vi "Test Attach Debugger.vi"   [LabVIEW 2020, in "Test Process.lvclass"]
uses:
  Test Process.lvclass
  C:/Program Files (x86)/National Instruments/LabVIEW 2020/vi.lib/Astemes/Triarc Framework/Process/Process.lvclass
  <vilib>/Astemes/Triarc Framework/Process/Process.lvclass/Process.ctl
  <vilib>/Astemes/Triarc Framework/Process/Private/SubVIs/Wait for finish.vi
  <vilib>/Astemes/Triarc Framework/Process/Protected/Messaging/Enqueue Message.vi
  <vilib>/Astemes/Triarc Framework/Process/Private/SubVIs/Set Lifecycle State.vi
  <vilib>/Astemes/Triarc Framework/Process/Public/Lifecycle/Get Lifecycle State.vi
  <vilib>/Astemes/Triarc Framework/Process/Private/SubVIs/Handle Debug Data.vi
  <vilib>/Utility/error.llb/Clear Errors.vi
  <vilib>/Astemes/Triarc Framework/Logging/Log Debug.vi
  <vilib>/AdvancedString/1D String Array to Delimited String.vi
  <vilib>/Utility/High Resolution Relative Seconds.vi
  <vilib>/Utility/error.llb/Error Cluster From Error Code.vi
  <vilib>/Astemes/Triarc Framework/Process/Public/Read Name.vi
  <vilib>/Astemes/Triarc Framework/Process/Process.lvclass
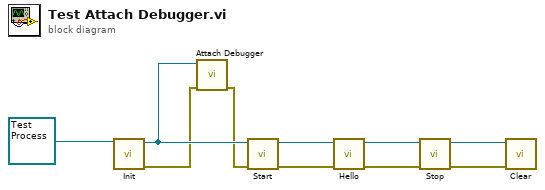
[diagram p0: block diagram]
diagram:
  n1 = call-dynamic "Init.vi"("Process In"=refnum<class "Test Process.lvclass"> refnum ("Test Process.lvclass")) -> ("error out"=w2:errorcluster, "Process Out"=w3:refnum<class "Test Process.lvclass">)  [unwired: 9 in]
  n2 = call "Attach Debugger.vi"("error in (no error)"=w2, "Process In"=w3) -> ("error out"=w1:errorcluster)  [unwired: 9 in]
  n3 = call <vilib>:"Start.vi"("error in (no error)"=w1, "Process In"=w3) -> ("error out"=w10:errorcluster, "Process Out"=w4:refnum<class "Test Process.lvclass">)  [unwired: 7 in, 1 out]
  n4 = call "Hello.vi"("error in (no error)"=w10, "Test Process In"=w4) -> ("error out"=w8:errorcluster, "Test Process Out"=w9:refnum<class "Test Process.lvclass">)  [unwired: 8 in]
  n5 = call <vilib>:"Stop.vi"("error in (no error)"=w8, "Process In"=w9) -> ("error out"=w6:errorcluster, "Process Out"=w7:refnum<class "Test Process.lvclass">)  [unwired: 7 in, 1 out]
  n6 = call-dynamic "Clear.vi"("error in (no error)"=w6, "Process In"=w7) -> ()  [unwired: 9 in, 1 out]
